vi "Cryo-Con Get Settigns.vi"(8 "Error In":errorcluster, 10 "Inputs":string[](array[string]), 11 "VISA resource name":refnum<visa-resource-name>) -> (0 "Error Out":errorcluster, 1 "Settings":string[](array[string]), 3 "VISA resource name out":refnum<visa-resource-name>)   [LabVIEW 2019]
uses:
  GPIB/VISA  Send Receive.vi
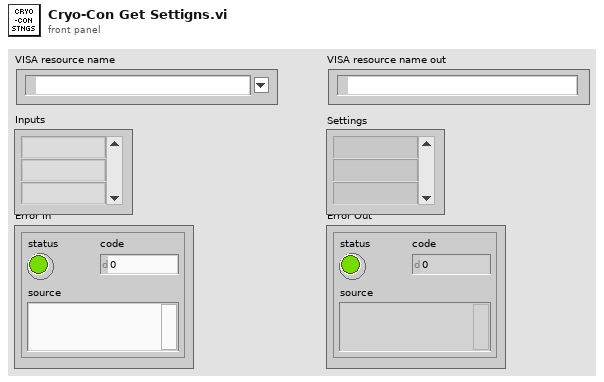
[diagram p1: front panel]
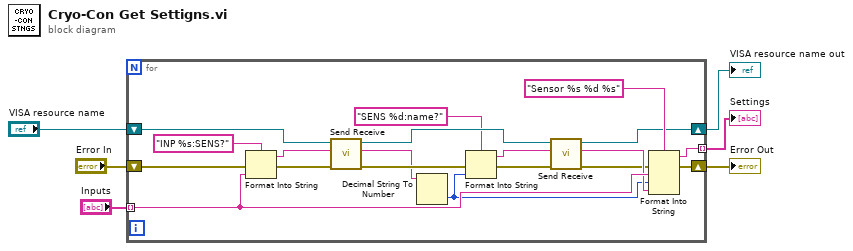
[diagram p0: block diagram]
diagram:
  n1 = for {
    shift-right: [w10] -> w2
    shift-left: "VISA resource name" -> [w25]
    shift-right: [w20] -> w3
    shift-left: "Error In" -> [w22]
    tunnel: "Inputs" -> [w18] mode=indexing
    tunnel: [w17] -> w4 mode=indexing
    n2 = Format Into String(format string="INP %s:SENS?", error in=w22, w18) -> (resulting string=w23:string, error out=w21:errorcluster)  [unwired: 1 in]
    n3 = call-poly "Send Receive.vi"("error in (no error)"=w21, "data string in"=w23, "VISA Resource Name"=w25) -> ("error out"=w15:errorcluster, "data string out"=w12:string, "VISA Resource Name Out"=w16:refnum<visa-resource-name>)  [unwired: 6 in]
    n4 = Decimal String To Number(string=w12) -> (number=w7:i32)  [unwired: 2 in, 1 out]
    n5 = Format Into String(format string="SENS %d:name?", error in=w15, w7) -> (resulting string=w8:string, error out=w14:errorcluster)  [unwired: 1 in]
    n6 = call-poly "Send Receive.vi"("error in (no error)"=w14, "data string in"=w8, "VISA Resource Name"=w16) -> ("error out"=w9:errorcluster, "data string out"=w11:string, "VISA Resource Name Out"=w10:refnum<visa-resource-name>)  [unwired: 6 in]
    n7 = Format Into String(format string="Sensor %s %d %s", error in=w9, w18, w7, w11) -> (resulting string=w17:string, error out=w20:errorcluster)  [unwired: 1 in]
  }
  "VISA resource name out" <- w2
  "Error Out" <- w3
  "Settings" <- w4
